vi "Service Mode Version Parse LE.vi"(0 "GEA2 Reference In":refnum<k24>, 5 "Version Selection":T1, 7 "Board ?":enum16{"UI", "MC"}(ring), 11 "Error In":errorcluster) -> (1 "Crit 1":string, 2 "Crit 2":string, 3 "Crit 3":string, 4 "GEA2 Reference Out":refnum<k24>, 6 "NonCrit 2":string, 8 "NonCrit 3":string, 10 "NonCrit 4":string, 12 "Crit 4":string, 13 "NonCrit 1":string, 15 "Error Out":errorcluster)   [LabVIEW 2016, in "Centauro.lvlib"]
uses:
  Projects/Centauro.lvlib
  Q:/Common/DLLs/GEA3/GeaCommunication.dll
  Common/DLLs/GEA3/GeaCommunication.dll
  type defs/Service Mode Version Selection.ctl
  Common/LabVIEW GEA2 Toolkit/LabVIEW_GEA2_Toolkit.lvlibp/type defs/ERD Read Data In.ctl
  Common/LabVIEW GEA2 Toolkit/LabVIEW_GEA2_Toolkit.lvlibp/type defs/Data Type.ctl
  Common/LabVIEW GEA2 Toolkit/LabVIEW_GEA2_Toolkit.lvlibp/type defs/Source_Destination.ctl
  Common/LabVIEW GEA2 Toolkit/LabVIEW_GEA2_Toolkit.lvlibp
panel:
  in  "Standalone?":bool
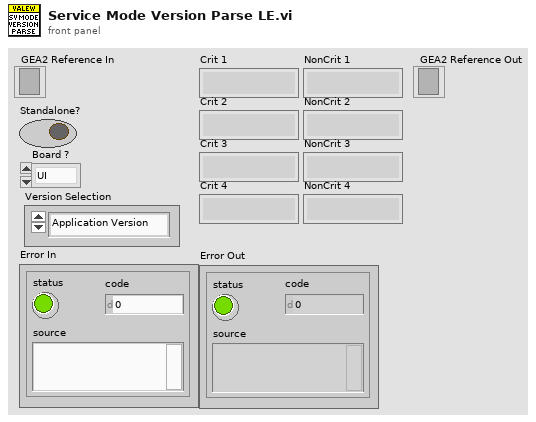
[diagram p1: front panel]
types:
  T1 = typedef "Centauro.lvlib/Service Mode Version Selection.ctl" = enum16{"Application Version", "XML Version"}
  T2 = typedef "LabVIEW_GEA2_Toolkit.lvlibp/ERD Read Data In.ctl" = cluster{"ERD Number":u16, "Data Type":T3}
  T3 = typedef "LabVIEW_GEA2_Toolkit.lvlibp/Data Type.ctl" = enum16{"string", "boolean", "uint8_t", "uint16_t", "uint32_t", "uint64_t", "int8_t", "int16_t", "int32_t", "int64_t"}
  T4 = typedef "LabVIEW_GEA2_Toolkit.lvlibp/Source_Destination.ctl" = cluster{"Source":u8, "Destination":u8}
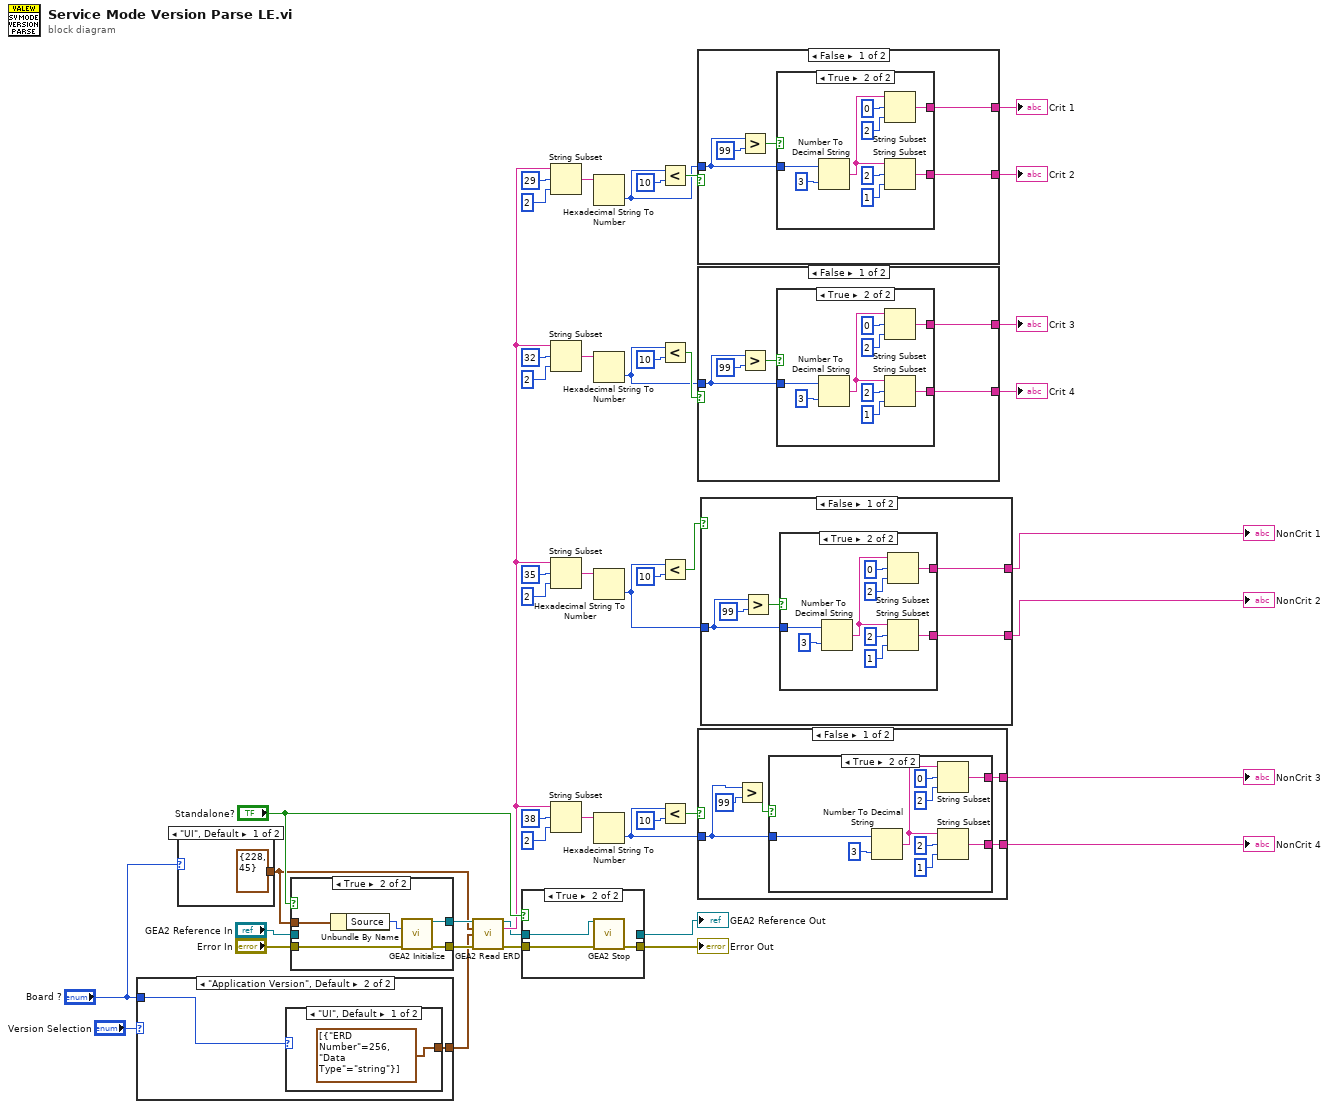
[diagram p0: block diagram]
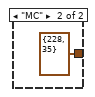
[diagram p2: hidden frame]
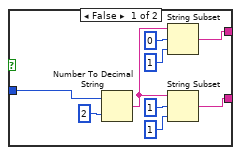
[diagram p3: hidden frame]
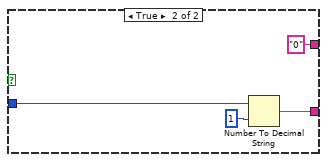
[diagram p4: hidden frame]
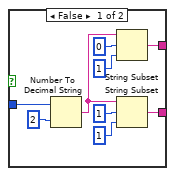
[diagram p5: hidden frame]
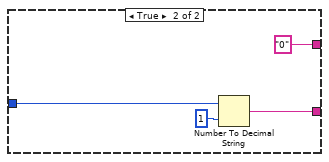
[diagram p6: hidden frame]
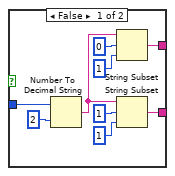
[diagram p7: hidden frame]
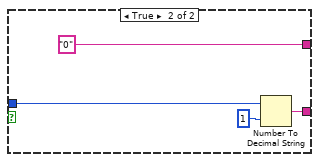
[diagram p8: hidden frame]
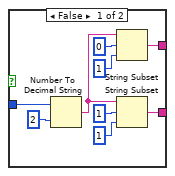
[diagram p9: hidden frame]
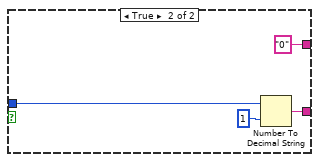
[diagram p10: hidden frame]
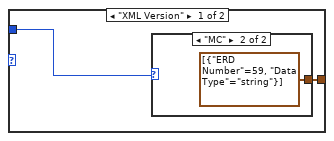
[diagram p11: hidden frame]
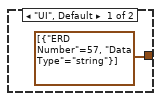
[diagram p12: hidden frame]
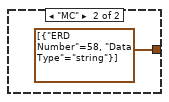
[diagram p13: hidden frame]
diagram:
  n1 = case shown="\"Application Version\", Default" "Version Selection" {
    tunnel: [w48 w52] -> w4
    tunnel: "Board ?" -> [w47 w51]
    frame "XML Version" {
      n2 = case shown="\"MC\"" w47 {
        tunnel: [T2[] [{"ERD Number"=57, "Data Type"=enum."string"}] ("Read ERD List") T2[] [{"ERD Number"=59, "Data Type"=enum."string"}] ("Read ERD List")] -> w48
        frame "UI", Default {
        }
        frame "MC" {
        }
      }
    }
    frame "Application Version", Default {
      n3 = case shown="\"UI\", Default" w51 {
        tunnel: [T2[] [{"ERD Number"=256, "Data Type"=enum."string"}] ("Read ERD List") T2[] [{"ERD Number"=58, "Data Type"=enum."string"}] ("Read ERD List")] -> w52
        frame "UI", Default {
        }
        frame "MC" {
        }
      }
    }
  }
  n4 = case shown="\"UI\", Default" "Board ?" {
    tunnel: [T4 {"Source"=228, "Destination"=45} ("GEA Inputs") T4 {"Source"=228, "Destination"=35} ("GEA Inputs")] -> w5
    frame "UI", Default {
    }
    frame "MC" {
    }
  }
  n5 = case shown="True" "Standalone?" {
    tunnel: "Error In" -> [w57 w63]
    tunnel: [w57 w62] -> w41
    tunnel: "GEA2 Reference In" -> [w58 _]
    tunnel: [w58 w61] -> w40
    tunnel: w5 -> [_ w59]
    frame False {
    }
    frame True {
      n6 = Unbundle By Name(w59) -> ("Source"=w60:u8)
      n7 = call "GEA2 Initialize.vi"("Source Address"=w60, "error in"=w63) -> ("GEA2 Reference Out"=w61:refnum<k24>, "error out"=w62:errorcluster)  [unwired: 11 in, 1 out]
    }
  }
  n8 = call "GEA2 Read ERD.vi"("GEA2 Reference In"=w40, "GEA Inputs"=w5, "Read ERD List"=w4, "Error In"=w41) -> ("GEA2 Reference Out"=w3:refnum<k24>, "Raw Data Out"=w30:string, "Error Out"=w2:errorcluster)  [unwired: 8 in, 1 out]
  n9 = case shown="True" "Standalone?" {
    tunnel: [w64 w68] -> w44
    tunnel: w3 -> [w65 w67]
    tunnel: [w65 _] -> w43
    tunnel: w2 -> [w64 w66]
    frame False {
    }
    frame True {
      n10 = call "GEA2 Stop.vi"("GEA2 Reference In"=w67, "Error In"=w66) -> ("Error Out"=w68:errorcluster)  [unwired: 13 in]
    }
  }
  "Error Out" <- w44
  "GEA2 Reference Out" <- w43
  n11 = String Subset(string=w30, offset (0)=29, length (rest)=2 ("length (rest)")) -> (substring=w29:string)
  n12 = String Subset(string=w30, offset (0)=32, length (rest)=2 ("length (rest)")) -> (substring=w28:string)
  n13 = String Subset(string=w30, offset (0)=35, length (rest)=2 ("length (rest)")) -> (substring=w27:string)
  n14 = String Subset(string=w30, offset (0)=38, length (rest)=2 ("length (rest)")) -> (substring=w26:string)
  n15 = Hexadecimal String To Number(string=w29) -> (number=w21:u32)  [unwired: 2 in, 1 out]
  n16 = Hexadecimal String To Number(string=w28) -> (number=w16:u32)  [unwired: 2 in, 1 out]
  n17 = Hexadecimal String To Number(string=w27) -> (number=w7:u32)  [unwired: 2 in, 1 out]
  n18 = Hexadecimal String To Number(string=w26) -> (number=w6:u32)  [unwired: 2 in, 1 out]
  n19 = Less?(x=w21, y=u32 10) -> (x < y?=w24:bool)
  n20 = Less?(x=w16, y=u32 10) -> (x < y?=w17:bool)
  n21 = Less?(x=w7, y=u32 10) -> (x < y?=w12:bool)
  n22 = Less?(x=w6, y=u32 10) -> (x < y?=w11:bool)
  n23 = case shown="False" w24 {
    tunnel: [w73 "0"] -> w22
    tunnel: w21 -> [w71 w93]
    tunnel: [w72 w92] -> w23
    frame False {
      n24 = Greater?(x=w71, y=u32 99) -> (0:w69:bool)
      n25 = case shown="True" w69 {
        tunnel: [w76 w87] -> w73
        tunnel: [w75 w86] -> w72
        tunnel: w71 -> [w77 w83]
        frame False {
          n26 = Number To Decimal String(number=w77, width (-)=i16 2) -> (decimal integer string=w82:string)
          n27 = String Subset(string=w82, offset (0)=0, length (rest)=1 ("length (rest)")) -> (substring=w76:string)
          n28 = String Subset(string=w82, offset (0)=1, length (rest)=1 ("length (rest)")) -> (substring=w75:string)
        }
        frame True {
          n29 = Number To Decimal String(number=w83, width (-)=i16 3) -> (decimal integer string=w90:string)
          n30 = String Subset(string=w90, offset (0)=0, length (rest)=2 ("length (rest)")) -> (substring=w87:string)
          n31 = String Subset(string=w90, offset (0)=2, length (rest)=1 ("length (rest)")) -> (substring=w86:string)
        }
      }
    }
    frame True {
      n32 = Number To Decimal String(number=w93, width (-)=i16 1) -> (decimal integer string=w92:string)
    }
  }
  "Crit 1" <- w22
  "Crit 2" <- w23
  n33 = case shown="False" w17 {
    tunnel: [w100 "0"] -> w20
    tunnel: w16 -> [w98 w120]
    tunnel: [w99 w119] -> w19
    frame False {
      n34 = Greater?(x=w98, y=u32 99) -> (0:w96:bool)
      n35 = case shown="True" w96 {
        tunnel: [w102 w114] -> w100
        tunnel: [w101 w113] -> w99
        tunnel: w98 -> [w103 w110]
        frame False {
          n36 = Number To Decimal String(number=w103, width (-)=i16 2) -> (decimal integer string=w109:string)
          n37 = String Subset(string=w109, offset (0)=0, length (rest)=1 ("length (rest)")) -> (substring=w102:string)
          n38 = String Subset(string=w109, offset (0)=1, length (rest)=1 ("length (rest)")) -> (substring=w101:string)
        }
        frame True {
          n39 = Number To Decimal String(number=w110, width (-)=i16 3) -> (decimal integer string=w117:string)
          n40 = String Subset(string=w117, offset (0)=0, length (rest)=2 ("length (rest)")) -> (substring=w114:string)
          n41 = String Subset(string=w117, offset (0)=2, length (rest)=1 ("length (rest)")) -> (substring=w113:string)
        }
      }
    }
    frame True {
      n42 = Number To Decimal String(number=w120, width (-)=i16 1) -> (decimal integer string=w119:string)
    }
  }
  "Crit 3" <- w20
  "Crit 4" <- w19
  n43 = case shown="False" w11 {
    tunnel: [w127 "0"] -> w8
    tunnel: w6 -> [w124 w147]
    tunnel: [w126 w146] -> w9
    frame False {
      n44 = Greater?(x=w124, y=u32 99) -> (0:w125:bool)
      n45 = case shown="True" w125 {
        tunnel: w124 -> [w128 w144]
        tunnel: [w130 w140] -> w127
        tunnel: [w129 w139] -> w126
        frame False {
          n46 = Number To Decimal String(number=w128, width (-)=i16 2) -> (decimal integer string=w131:string)
          n47 = String Subset(string=w131, offset (0)=0, length (rest)=1 ("length (rest)")) -> (substring=w130:string)
          n48 = String Subset(string=w131, offset (0)=1, length (rest)=1 ("length (rest)")) -> (substring=w129:string)
        }
        frame True {
          n49 = Number To Decimal String(number=w144, width (-)=i16 3) -> (decimal integer string=w143:string)
          n50 = String Subset(string=w143, offset (0)=0, length (rest)=2 ("length (rest)")) -> (substring=w140:string)
          n51 = String Subset(string=w143, offset (0)=2, length (rest)=1 ("length (rest)")) -> (substring=w139:string)
        }
      }
    }
    frame True {
      n52 = Number To Decimal String(number=w147, width (-)=i16 1) -> (decimal integer string=w146:string)
    }
  }
  "NonCrit 3" <- w8
  "NonCrit 4" <- w9
  n53 = case shown="False" w12 {
    tunnel: [w154 "0"] -> w15
    tunnel: w7 -> [w151 w174]
    tunnel: [w153 w173] -> w14
    frame False {
      n54 = Greater?(x=w151, y=u32 99) -> (0:w152:bool)
      n55 = case shown="True" w152 {
        tunnel: w151 -> [w156 w171]
        tunnel: [w158 w167] -> w154
        tunnel: [w155 w166] -> w153
        frame False {
          n56 = Number To Decimal String(number=w156, width (-)=i16 2) -> (decimal integer string=w157:string)
          n57 = String Subset(string=w157, offset (0)=0, length (rest)=1 ("length (rest)")) -> (substring=w158:string)
          n58 = String Subset(string=w157, offset (0)=1, length (rest)=1 ("length (rest)")) -> (substring=w155:string)
        }
        frame True {
          n59 = Number To Decimal String(number=w171, width (-)=i16 3) -> (decimal integer string=w170:string)
          n60 = String Subset(string=w170, offset (0)=0, length (rest)=2 ("length (rest)")) -> (substring=w167:string)
          n61 = String Subset(string=w170, offset (0)=2, length (rest)=1 ("length (rest)")) -> (substring=w166:string)
        }
      }
    }
    frame True {
      n62 = Number To Decimal String(number=w174, width (-)=i16 1) -> (decimal integer string=w173:string)
    }
  }
  "NonCrit 1" <- w15
  "NonCrit 2" <- w14
